vi "Get name from configuration.vi"(0 "Configuration":T1, 1 "Type":string) -> (7 "Name":string, 8 "Found?":bool)   [LabVIEW 2014]
uses:
  Configuration.ctl
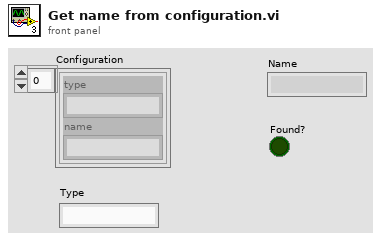
[diagram p1: front panel]
types:
  T1 = typedef "Configuration.ctl" = cluster{"type":string, "name":string}[]
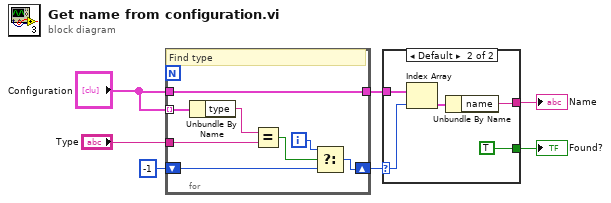
[diagram p0: block diagram]
diagram:
  n1 = for {
    tunnel: "Configuration" -> [w15] mode=indexing
    tunnel: "Type" -> [w13]
    shift-right: [w11] -> w5
    shift-left: -1 -> [w9]
    tunnel: [w8] -> w4
    tunnel: "Configuration" -> [w8]
    i -> [w10]
    # "Find type"
    n2 = Unbundle By Name(w15) -> ("type"=w14:string)
    n3 = Equal?(x=w14, y=w13) -> (x = y?=w12:bool)
    n4 = Select(t=w10, s=w12, f=w9) -> (s? t:f=w11:i32)
  }
  n5 = case shown="Default" w5 {
    selector: w5 -> [_ w20]
    tunnel: w4 -> [_ w19]
    tunnel: [_ w17] -> w3
    tunnel: [_ TRUE] -> w2
    frame -1 {
    }
    frame Default {
      n6 = Index Array(array=w19, index=w20) -> (element=w18:cluster{"type":string, "name":string})
      n7 = Unbundle By Name(w18) -> ("name"=w17:string)
    }
  }
  "Name" <- w3
  "Found?" <- w2
